vi "SetHostName.vi"(4 "error in (no error)":errorcluster, 5 "Hostname":string, 6 "DeviceKey In":string, 7 "CmdLib In":refnum<k24>) -> (0 "error out":errorcluster, 2 "DeviceKey Out":string, 3 "CmdLib Out":refnum<k24>)   [LabVIEW 2009]
uses:
  C:/Code/Apps/Utilities/Picomotor/PicomotorApp/Install/Samples/LabVIEW/Model 8742/LabVIEW 2009/CmdLib.dll
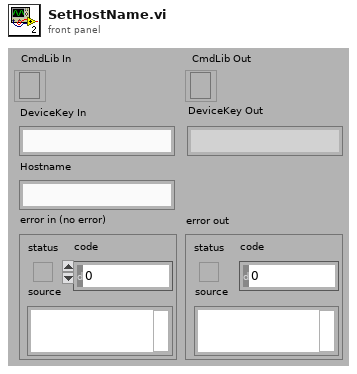
[diagram p1: front panel]
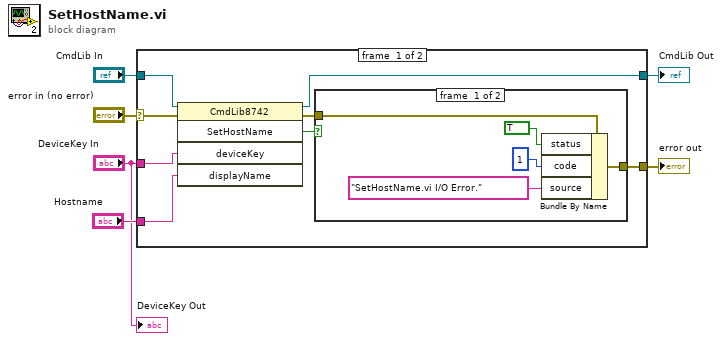
[diagram p0: block diagram]
diagram:
  n1 = case shown="No Error" "error in (no error)" {
    selector: "error in (no error)" -> [w10 w21]
    tunnel: "CmdLib In" -> [w14 w22]
    tunnel: [w13 w22] -> w5
    tunnel: "Hostname" -> [w12 _]
    tunnel: "DeviceKey In" -> [w11 _]
    tunnel: [w7 w21] -> w1
    frame #0 {
      n2 = invoke class="CmdLib8742" method="SetHostName"(reference=w14, error in=w10, "deviceKey"=w11, "displayName"=w12) -> (reference out=w13:refnum<k24>, error out=w8:errorcluster, "SetHostName"=w9:bool)  [unwired: 1 in, 2 out]
      n3 = case shown="False" w9 {
        tunnel: w8 -> [w19 w20]
        tunnel: [w18 w20] -> w7
        frame #0 {
          n4 = Bundle By Name(cluster=w19, "status"=TRUE, "code"=1, "source"="SetHostName.vi I/O Error.") -> (w18:errorcluster)
        }
        frame #1 {
        }
      }
    }
    frame #1 {
    }
  }
  "error out" <- w1
  "CmdLib Out" <- w5
  "DeviceKey Out" <- "DeviceKey In"
